vi "Detector Get Image.vi"(8 "error in (no error)":errorcluster, 10 "Observation":T1={"Priority"=0, "ID"="", "Observer"="", "Obj Name"="", "Obj Type"="", "RA and DEC String"={"RA"="HH:MM:SS.nnn", "DEC"="DEG:arcmin:arcsec.nn"}, "Filters"=[], "Integration Time"=0.0, "Observation Status"=enum."Error", "Offsets"={"RA"=0.0, "DEC"=0.0, "ROT"=0.0}, "Images"=0, "Dither Options"={"Dither"=enum."None", "Dither Radius"=0.0, "Dither Points"=0, "Dither Phase"=0.0, "B Offset"={"RA"=0.0, "DEC"=0.0}}, "Comment 1"="", "Comment 2"=""}, 11 "PRIME Detector in":refnum<class "PRIME Detector.lvclass">) -> (0 "error out":errorcluster, 1 "FITS Detector Settings":T8, 2 "Images":T9[](array[typedef]), 3 "PRIME Detector out":refnum<class "PRIME Detector.lvclass">, 4 "Message Log":string, 6 "Detector Files":T7)   [LabVIEW 2024, in "PRIME Detector.lvclass"]
uses:
  PRIME Detector.lvclass
  Detector Image typedef cluster.ctl
  RIMAS Observation Config.ctl
  Detector cluster Files.ctl
  typedefs/CC cluster Observation.ctl
  Observation Queue/CC enum Observation Status.ctl
  Telescope/CC cluster Telescope Offsets.ctl
  typedefs/CC cluster Observation Dither Options.ctl
  typedefs/CC enum Dither Selection.ctl
  typedefs/CC cluster RA and DEC.ctl
  Detector Class.lvclass
  PRIME Detector.lvclass/PRIME Detector.ctl
  ed270338-c6d5-43e5-a287-b31ed10c4701.vi
  81b43f0d-8b71-4fcf-9938-3437e86aa932.vi
panel:
  out "Table":string[](array[string])
  # "Make sure that the timeout is set to exceed the maximal exposure time, otherwise the acuisition fails"
  # "sec"
  # "sec"
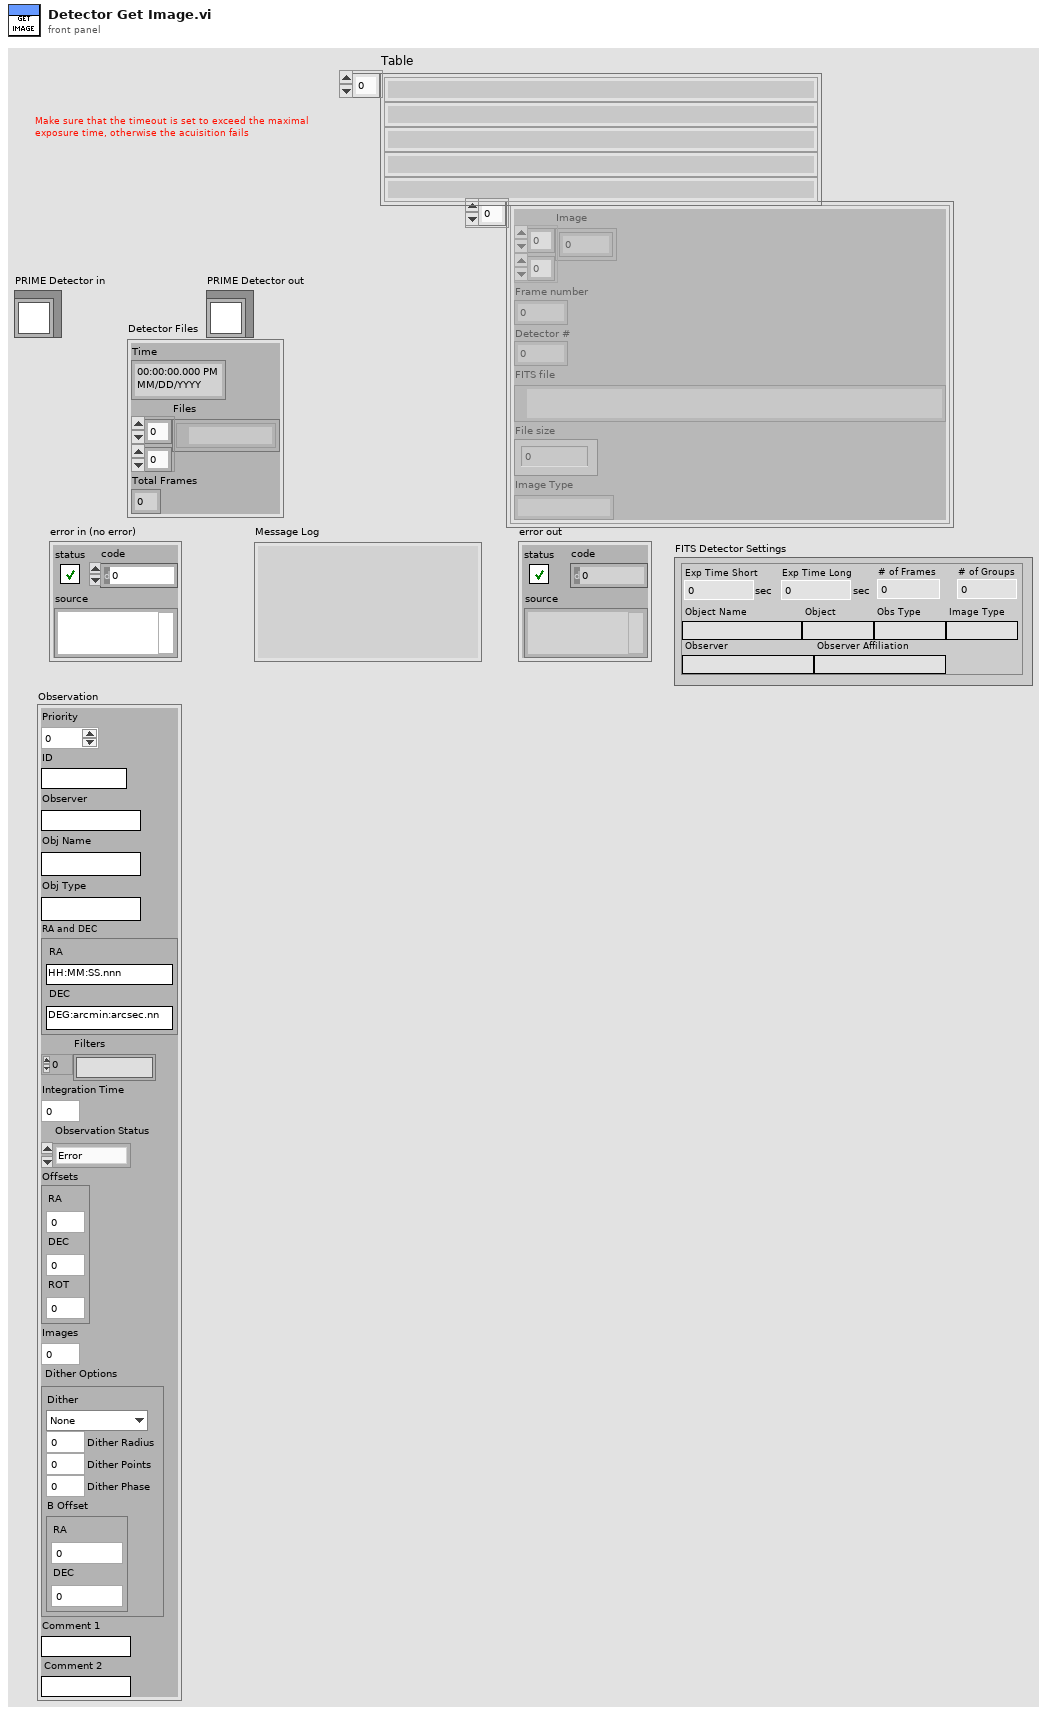
[diagram p1: front panel]
types:
  T1 = typedef "CC cluster Observation.ctl" = cluster{"Priority":i32, "ID":string, "Observer":string, "Obj Name":string, "Obj Type":string, "RA and DEC String":cluster{"RA":string, "DEC":string}, "Filters":string[], "Integration Time":dbl, "Observation Status":T2, "Offsets":T3, "Images":i32, "Dither Options":T4, "Comment 1":string, "Comment 2":string}
  T2 = typedef "CC enum Observation Status.ctl" = enum16{"Ready", "Running", "Done", "Error"}
  T3 = typedef "CC cluster Telescope Offsets.ctl" = cluster{"RA":dbl, "DEC":dbl, "ROT":dbl}
  T4 = typedef "CC cluster Observation Dither Options.ctl" = cluster{"Dither":T5, "Dither Radius":dbl, "Dither Points":i32, "Dither Phase":dbl, "B Offset":T6}
  T5 = typedef "CC enum Dither Selection.ctl" = enum16{"None", "Circle", "Random", "ABBA"}
  T6 = typedef "CC cluster RA and DEC.ctl" = cluster{"RA":dbl, "DEC":dbl}
  T7 = typedef "Detector Class.lvclass/Detector cluster Files.ctl" = cluster{"Time":timestamp, "Files":path[][], "Total Frames":i32}
  T8 = typedef "RIMAS Observation Config.ctl" = cluster{"Exp Time Short":dbl, "# of Frames":dbl, "Exp Time Long":dbl, "# of Groups":dbl, "Object Name":string, "Object":string, "Obs Type":string, "Image Type":string, "Observer":string, "Observer Affiliation":string}
  T9 = typedef "Detector Class.lvclass/Detector Image typedef cluster.ctl" = cluster{"Image":sgl[][], "Frame number":i32, "Detector #":u16, "FITS file":path, "File size":i64, "Image Type":string}
  T10 = typedef "RIMAS Detector Config.ctl" = cluster{"Detector":u16, "Offsets":u16[][], "Detector Computer":T11, "FITS hdr template0":path, "FITS hdr template1":path, "FITS Data File Path":path, "FITS Detector Settings":T8, "Sim Folder":path, "Integration Mode":T12, "Integration Time":dbl, "Frame Int Time":dbl}
  T11 = typedef "RIMAS Detector Server Config.ctl" = cluster{"Machine":string, "Password":string, "FITS File Path":string, "Port":u16, "Header Path":string, "Name":string}
  T12 = typedef "Detector enum Detector Integration Mode.ctl" = enum16{"Ramp", "CDS", "FOWLER2", "FOWLER4", "FOWLER8", "FOWLER16", "Raw"}
  T13 = typedef "PRIME Detector cluster Status.ctl" = cluster{"Cmd Start Time":timestamp, "Command":string, "Complete?":bool, "Cmd Complete Time":timestamp, "Exp Time Remaining":dbl, "Total Frames":i32, "Exp Frames":cluster{"CAMERA0":string[], "CAMERA1":string[], "CAMERA2":string[], "CAMERA3":string[]}, "Intermediate Frames":cluster{"CAMERA0":string[], "CAMERA1":string[], "CAMERA2":string[], "CAMERA3":string[]}, "Final Reduced Frame":cluster{"CAMERA0":string, "CAMERA1":string, "CAMERA2":string, "CAMERA3":string}}
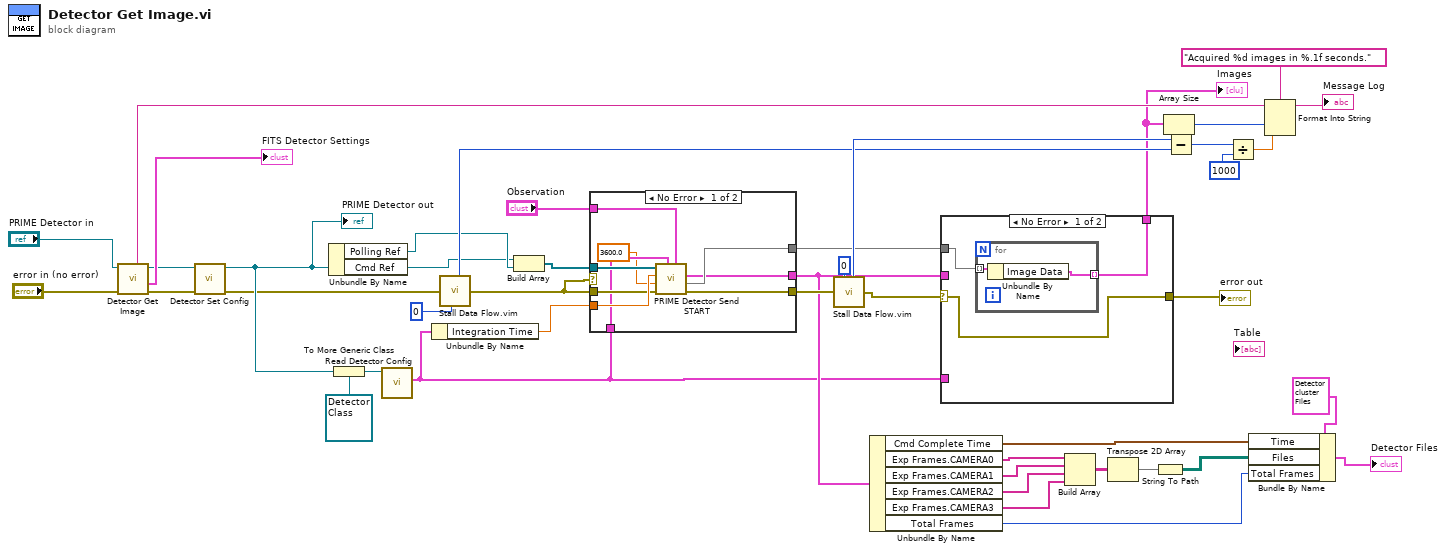
[diagram p0: block diagram]
diagram:
  n1 = call-parent "Detector Get Image.vi"("error in (no error)"="error in (no error)", "Detector Class in"="PRIME Detector in") -> ("error out"=w2:errorcluster, "FITS Detector Settings"=→"FITS Detector Settings":T8, "Detector Class out"=w4:refnum<class "PRIME Detector.lvclass">, "Message Log"=w31:string)  [unwired: 4 in, 2 out]
  n2 = call-dynamic "Detector Set Config.vi"("error in (no error)"=w2, "PRIME Detector in"=w4) -> ("error out"=w1:errorcluster, "PRIME Detector out"=w3:refnum<class "PRIME Detector.lvclass">)  [unwired: 8 in]
  "PRIME Detector out" <- w3
  n3 = Unbundle By Name(w3) -> ("Polling Ref"=w27:refnum<k5>, "Cmd Ref"=w21:refnum<k5>)
  n4 = To More Generic Class(target class=refnum<class "Detector Class.lvclass"> refnum ("Detector Class.lvclass"), reference=w3) -> (generic class reference=w41:refnum<class "Detector Class.lvclass">)
  n5 = call-dynamic "Read Detector Config.vi"("Detector Class in"=w41) -> ("Detector Config"=w6:T10)  [unwired: 8 in, 2 out]
  n6 = Unbundle By Name(w6) -> ("Integration Time"=w28:dbl)
  n7 = call "Stall Data Flow.vim"("value in"=w1, "milliseconds to wait"=u32 0) -> ("millisecond timer value"=w38:u32, "value out"=w20:errorcluster)
  n8 = Build Array(w21, w27) -> (w26:refnum<k5>[])
  n9 = case shown="No Error" w20 {
    tunnel: w28 -> [w53 _]
    tunnel: [w48 _] -> w14
    tunnel: w20 -> [w52 w54]
    tunnel: w26 -> [w51 _]
    tunnel: [w50 w54] -> w24
    tunnel: [w49 _] -> w7
    tunnel: w6 -> [w47 _]
    tunnel: "Observation" -> [w46 _]
    frame No Error {
      n10 = call "PRIME Detector Send START.vi"("Observation"=w46, "Detector Config"=w47, "error in (no error)"=w52, "timeout (120s)"=3600.0, "Exposure Time"=w53, "connection ID"=w51) -> ("error out"=w50:errorcluster, "Image Map"=w49:map{string, T9}, "Status out"=w48:T13)  [unwired: 2 in, 1 out]
    }
    frame Error {
    }
  }
  n11 = call "Stall Data Flow.vim"("value in"=w24, "milliseconds to wait"=u32 0) -> ("millisecond timer value"=w39:u32, "value out"=w22:errorcluster)
  n12 = Unbundle By Name(w14) -> ("Cmd Complete Time"=w12:timestamp, "Exp Frames.CAMERA0"=w19:string[], "Exp Frames.CAMERA1"=w18:string[], "Exp Frames.CAMERA2"=w17:string[], "Exp Frames.CAMERA3"=w16:string[], "Total Frames"=w11:i32)
  n13 = case shown="No Error" w22 {
    selector: w22 -> [w55 w60]
    tunnel: w6 -> [_ _]
    tunnel: [w56 _] -> w29
    tunnel: w14 -> [_ _]
    tunnel: [w55 w60] -> w23
    tunnel: w7 -> [w57 _]
    frame No Error {
      n14 = for {
        tunnel: w57 -> [w59] mode=indexing
        tunnel: [w58] -> w56 mode=indexing
        n15 = Unbundle By Name(w59) -> ("Image Data"=w58:T9)
      }
    }
    frame Error {
    }
  }
  "error out" <- w23
  "Images" <- w29
  n16 = Build Array(w19, w18, w17, w16) -> (w15:string[][])
  n17 = Transpose 2D Array(2D array=w15) -> (transposed array=w10:string[][])
  n18 = String To Path(string=w10) -> (path=w9:path[][])
  n19 = Array Size(array=w29) -> (size(s)=w36:i32)
  n20 = Subtract(x=w39, y=w38) -> (x-y=w35:u32)
  n21 = Divide(x=w35, y=u32 1000) -> (x/y=w33:dbl)
  n22 = Bundle By Name(cluster=T7 {"Time"=timestamp(0 s since 1904-01-01), "Files"=[], "Total Frames"=0} ("Detector Files"), "Time"=w12, "Files"=w9, "Total Frames"=w11) -> (→"Detector Files":T7)
  n23 = Format Into String(format string="Acquired %d images in %.1f seconds.", initial string=w31, w36, w33) -> (resulting string=→"Message Log":string)  [unwired: 1 in, 1 out]
